vi "子VI-计算框中心XY坐标值.vi"(11 "Global Rectangle":i32[](array[numeric])) -> (1 "中心Y":dbl, 3 "中心X":dbl)   [LabVIEW 2018]
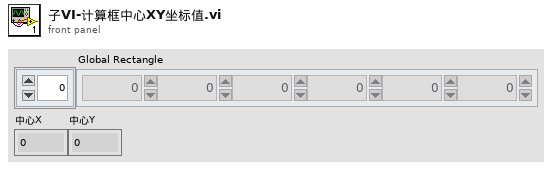
[diagram p1: front panel]
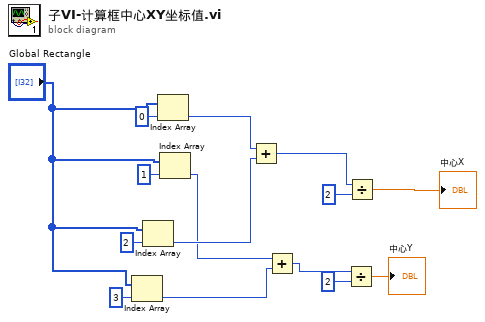
[diagram p0: block diagram]
diagram:
  n1 = Index Array(array="Global Rectangle", index=3 ("索引")) -> (element=w5:i32)
  n2 = Index Array(array="Global Rectangle", index=2 ("索引")) -> (element=w10:i32)
  n3 = Index Array(array="Global Rectangle", index=0 ("索引")) -> (element=w11:i32)
  n4 = Index Array(array="Global Rectangle", index=1 ("索引")) -> (element=w6:i32)
  n5 = Add(x=w11, y=w10) -> (x+y=w9:i32)
  n6 = Add(x=w6, y=w5) -> (x+y=w4:i32)
  n7 = Divide(x=w4, y=2) -> (x/y=→"中心Y":dbl)
  n8 = Divide(x=w9, y=2) -> (x/y=→"中心X":dbl)
